vi "App - analyze RUS V6.vi"() -> ()   [LabVIEW 2021] (continued)
(VHz)"=0.0, "ω (Hz)"=0.0, "Γ (Hz)"=0.0, "φ (rad)"=0.0, "Q"=0.0, "Norm  Ampl"=0.0, "z∞ (V)"=0.0+0.0i, "4corners"={"z (-pi/2)"=0.0+0.0i, "z(inf)"=0.0+0.0i, "z (pi/2)"=0.0+0.0i, "z center"=0.0+0.0i, "z(0)"=0.0+0.0i, "radius"=0.0}}, "timestamp(min)"=1041.0333333313465, "timestamp"=timestamp(3493790283 s since 1904-01-01), "Magn Field(T)"=0.0}, {"temperature"=68.294, "lorentzian"={"A (VHz)"=0.0, "ω (Hz)"=0.0, "Γ (Hz)"=0.0, "φ (rad)"=0.0, "Q"=0.0, "Norm  Ampl"=0.0, "z∞ (V)"=0.0+0.0i, "4corners"={"z (-pi/2)"=0.0+0.0i, "z(inf)"=0.0+0.0i, "z (pi/2)"=0.0+0.0i, "z center"=0.0+0.0i, "z(0)"=0.0+0.0i, "radius"=0.0}}, "timestamp(min)"=1042.3500000014901, "timestamp"=timestamp(3493790362 s since 1904-01-01), "Magn Field(T)"=0.0}, {"temperature"=68.232, "lorentzian"={"A (VHz)"=0.0, "ω (Hz)"=0.0, "Γ (Hz)"=0.0, "φ (rad)"=0.0, "Q"=0.0, "Norm  Ampl"=0.0, "z∞ (V)"=0.0+0.0i, "4corners"={"z (-pi/2)"=0.0+0.0i, "z(inf)"=0.0+0.0i, "z (pi/2)"=0.0+0.0i, "z center"=0.0+0.0i, "z(0)"=0.0+0.0i, "radius"=0.0}}, "timestamp(min)"=1043.683333337307, "timestamp"=timestamp(3493790442 s since 1904-01-01), "Magn Field(T)"=0.0}, {"temperature"=68.168, "lorentzian"={"A (VHz)"=0.0, "ω (Hz)"=0.0, "Γ (Hz)"=0.0, "φ (rad)"=0.0, "Q"=0.0, "Norm  Ampl"=0.0, "z∞ (V)"=0.0+0.0i, "4corners"={"z (-pi/2)"=0.0+0.0i, "z(inf)"=0.0+0.0i, "z (pi/2)"=0.0+0.0i, "z center"=0.0+0.0i, "z(0)"=0.0+0.0i, "radius"=0.0}}, "timestamp(min)"=1045.0, "timestamp"=timestamp(3493790521 s since 1904-01-01), "Magn Field(T)"=0.0}, {"temperature"=68.111, "lorentzian"={"A (VHz)"=0.0, "ω (Hz)"=0.0, "Γ (Hz)"=0.0, "φ (rad)"=0.0, "Q"=0.0, "Norm  Ampl"=0.0, "z∞ (V)"=0.0+0.0i, "4corners"={"z (-pi/2)"=0.0+0.0i, "z(inf)"=0.0+0.0i, "z (pi/2)"=0.0+0.0i, "z center"=0.0+0.0i, "z(0)"=0.0+0.0i, "radius"=0.0}}, "timestamp(min)"=1046.3166666701436, "timestamp"=timestamp(3493790600 s since 1904-01-01), "Magn Field(T)"=0.0}, {"temperature"=68.048, "lorentzian"={"A (VHz)"=0.0, "ω (Hz)"=0.0, "Γ (Hz)"=0.0, "φ (rad)"=0.0, "Q"=0.0, "Norm  Ampl"=0.0, "z∞ (V)"=0.0+0.0i, "4corners"={"z (-pi/2)"=0.0+0.0i, "z(inf)"=0.0+0.0i, "z (pi/2)"=0.0+0.0i, "z center"=0.0+0.0i, "z(0)"=0.0+0.0i, "radius"=0.0}}, "timestamp(min)"=1047.6499999985099, "timestamp"=timestamp(3493790680 s since 1904-01-01), "Magn Field(T)"=0.0}, {"temperature"=67.989, "lorentzian"={"A (VHz)"=0.0, "ω (Hz)"=0.0, "Γ (Hz)"=0.0, "φ (rad)"=0.0, "Q"=0.0, "Norm  Ampl"=0.0, "z∞ (V)"=0.0+0.0i, "4corners"={"z (-pi/2)"=0.0+0.0i, "z(inf)"=0.0+0.0i, "z (pi/2)"=0.0+0.0i, "z center"=0.0+0.0i, "z(0)"=0.0+0.0i, "radius"=0.0}}, "timestamp(min)"=1048.9666666686535, "timestamp"=timestamp(3493790759 s since 1904-01-01), "Magn Field(T)"=0.0}, {"temperature"=67.927, "lorentzian"={"A (VHz)"=0.0, "ω (Hz)"=0.0, "Γ (Hz)"=0.0, "φ (rad)"=0.0, "Q"=0.0, "Norm  Ampl"=0.0, "z∞ (V)"=0.0+0.0i, "4corners"={"z (-pi/2)"=0.0+0.0i, "z(inf)"=0.0+0.0i, "z (pi/2)"=0.0+0.0i, "z center"=0.0+0.0i, "z(0)"=0.0+0.0i, "radius"=0.0}}, "timestamp(min)"=1050.2833333313465, "timestamp"=timestamp(3493790838 s since 1904-01-01), "Magn Field(T)"=0.0}, {"temperature"=67.865, "lorentzian"={"A (VHz)"=0.0, "ω (Hz)"=0.0, "Γ (Hz)"=0.0, "φ (rad)"=0.0, "Q"=0.0, "Norm  Ampl"=0.0, "z∞ (V)"=0.0+0.0i, "4corners"={"z (-pi/2)"=0.0+0.0i, "z(inf)"=0.0+0.0i, "z (pi/2)"=0.0+0.0i, "z center"=0.0+0.0i, "z(0)"=0.0+0.0i, "radius"=0.0}}, "timestamp(min)"=1051.6166666671634, "timestamp"=timestamp(3493790918 s since 1904-01-01), "Magn Field(T)"=0.0}, {"temperature"=67.806, "lorentzian"={"A (VHz)"=0.0, "ω (Hz)"=0.0, "Γ (Hz)"=0.0, "φ (rad)"=0.0, "Q"=0.0, "Norm  Ampl"=0.0, "z∞ (V)"=0.0+0.0i, "4corners"={"z (-pi/2)"=0.0+0.0i, "z(inf)"=0.0+0.0i, "z (pi/2)"=0.0+0.0i, "z center"=0.0+0.0i, "z(0)"=0.0+0.0i, "radius"=0.0}}, "timestamp(min)"=1052.933333337307, "timestamp"=timestamp(3493790997 s since 1904-01-01), "Magn Field(T)"=0.0}, {"temperature"=67.745, "lorentzian"={"A (VHz)"=0.0, "ω (Hz)"=0.0, "Γ (Hz)"=0.0, "φ (rad)"=0.0, "Q"=0.0, "Norm  Ampl"=0.0, "z∞ (V)"=0.0+0.0i, "4corners"={"z (-pi/2)"=0.0+0.0i, "z(inf)"=0.0+0.0i, "z (pi/2)"=0.0+0.0i, "z center"=0.0+0.0i, "z(0)"=0.0+0.0i, "radius"=0.0}}, "timestamp(min)"=1054.2666666656733, "timestamp"=timestamp(3493791077 s since 1904-01-01), "Magn Field(T)"=0.0}, {"temperature"=67.683, "lorentzian"={"A (VHz)"=0.0, "ω (Hz)"=0.0, "Γ (Hz)"=0.0, "φ (rad)"=0.0, "Q"=0.0, "Norm  Ampl"=0.0, "z∞ (V)"=0.0+0.0i, "4corners"={"z (-pi/2)"=0.0+0.0i, "z(inf)"=0.0+0.0i, "z (pi/2)"=0.0+0.0i, "z center"=0.0+0.0i, "z(0)"=0.0+0.0i, "radius"=0.0}}, "timestamp(min)"=1055.5833333358169, "timestamp"=timestamp(3493791156 s since 1904-01-01), "Magn Field(T)"=0.0}, {"temperature"=67.625, "lorentzian"={"A (VHz)"=0.0, "ω (Hz)"=0.0, "Γ (Hz)"=0.0, "φ (rad)"=0.0, "Q"=0.0, "Norm  Ampl"=0.0, "z∞ (V)"=0.0+0.0i, "4corners"={"z (-pi/2)"=0.0+0.0i, "z(inf)"=0.0+0.0i, "z (pi/2)"=0.0+0.0i, "z center"=0.0+0.0i, "z(0)"=0.0+0.0i, "radius"=0.0}}, "timestamp(min)"=1056.8999999985099, "timestamp"=timestamp(3493791235 s since 1904-01-01), "Magn Field(T)"=0.0}, {"temperature"=67.561, "lorentzian"={"A (VHz)"=0.0, "ω (Hz)"=0.0, "Γ (Hz)"=0.0, "φ (rad)"=0.0, "Q"=0.0, "Norm  Ampl"=0.0, "z∞ (V)"=0.0+0.0i, "4corners"={"z (-pi/2)"=0.0+0.0i, "z(inf)"=0.0+0.0i, "z (pi/2)"=0.0+0.0i, "z center"=0.0+0.0i, "z(0)"=0.0+0.0i, "radius"=0.0}}, "timestamp(min)"=1058.2333333343267, "timestamp"=timestamp(3493791315 s since 1904-01-01), "Magn Field(T)"=0.0}, {"temperature"=67.503, "lorentzian"={"A (VHz)"=0.0, "ω (Hz)"=0.0, "Γ (Hz)"=0.0, "φ (rad)"=0.0, "Q"=0.0, "Norm  Ampl"=0.0, "z∞ (V)"=0.0+0.0i, "4corners"={"z (-pi/2)"=0.0+0.0i, "z(inf)"=0.0+0.0i, "z (pi/2)"=0.0+0.0i, "z center"=0.0+0.0i, "z(0)"=0.0+0.0i, "radius"=0.0}}, "timestamp(min)"=1059.5500000044703, "timestamp"=timestamp(3493791394 s since 1904-01-01), "Magn Field(T)"=0.0}, {"temperature"=67.441, "lorentzian"={"A (VHz)"=0.0, "ω (Hz)"=0.0, "Γ (Hz)"=0.0, "φ (rad)"=0.0, "Q"=0.0, "Norm  Ampl"=0.0, "z∞ (V)"=0.0+0.0i, "4corners"={"z (-pi/2)"=0.0+0.0i, "z(inf)"=0.0+0.0i, "z (pi/2)"=0.0+0.0i, "z center"=0.0+0.0i, "z(0)"=0.0+0.0i, "radius"=0.0}}, "timestamp(min)"=1060.8666666671634, "timestamp"=timestamp(3493791473 s since 1904-01-01), "Magn Field(T)"=0.0}, {"temperature"=67.379, "lorentzian"={"A (VHz)"=0.0, "ω (Hz)"=0.0, "Γ (Hz)"=0.0, "φ (rad)"=0.0, "Q"=0.0, "Norm  Ampl"=0.0, "z∞ (V)"=0.0+0.0i, "4corners"={"z (-pi/2)"=0.0+0.0i, "z(inf)"=0.0+0.0i, "z (pi/2)"=0.0+0.0i, "z center"=0.0+0.0i, "z(0)"=0.0+0.0i, "radius"=0.0}}, "timestamp(min)"=1062.2000000029802, "timestamp"=timestamp(3493791553 s since 1904-01-01), "Magn Field(T)"=0.0}, {"temperature"=67.322, "lorentzian"={"A (VHz)"=0.0, "ω (Hz)"=0.0, "Γ (Hz)"=0.0, "φ (rad)"=0.0, "Q"=0.0, "Norm  Ampl"=0.0, "z∞ (V)"=0.0+0.0i, "4corners"={"z (-pi/2)"=0.0+0.0i, "z(inf)"=0.0+0.0i, "z (pi/2)"=0.0+0.0i, "z center"=0.0+0.0i, "z(0)"=0.0+0.0i, "radius"=0.0}}, "timestamp(min)"=1063.5166666656733, "timestamp"=timestamp(3493791632 s since 1904-01-01), "Magn Field(T)"=0.0}, {"temperature"=67.261, "lorentzian"={"A (VHz)"=0.0, "ω (Hz)"=0.0, "Γ (Hz)"=0.0, "φ (rad)"=0.0, "Q"=0.0, "Norm  Ampl"=0.0, "z∞ (V)"=0.0+0.0i, "4corners"={"z (-pi/2)"=0.0+0.0i, "z(inf)"=0.0+0.0i, "z (pi/2)"=0.0+0.0i, "z center"=0.0+0.0i, "z(0)"=0.0+0.0i, "radius"=0.0}}, "timestamp(min)"=1064.8333333358169, "timestamp"=timestamp(3493791711 s since 1904-01-01), "Magn Field(T)"=0.0}, {"temperature"=67.202, "lorentzian"={"A (VHz)"=0.0, "ω (Hz)"=0.0, "Γ (Hz)"=0.0, "φ (rad)"=0.0, "Q"=0.0, "Norm  Ampl"=0.0, "z∞ (V)"=0.0+0.0i, "4corners"={"z (-pi/2)"=0.0+0.0i, "z(inf)"=0.0+0.0i, "z (pi/2)"=0.0+0.0i, "z center"=0.0+0.0i, "z(0)"=0.0+0.0i, "radius"=0.0}}, "timestamp(min)"=1066.1666666641831, "timestamp"=timestamp(3493791791 s since 1904-01-01), "Magn Field(T)"=0.0}, {"temperature"=67.139, "lorentzian"={"A (VHz)"=0.0, "ω (Hz)"=0.0, "Γ (Hz)"=0.0, "φ (rad)"=0.0, "Q"=0.0, "Norm  Ampl"=0.0, "z∞ (V)"=0.0+0.0i, "4corners"={"z (-pi/2)"=0.0+0.0i, "z(inf)"=0.0+0.0i, "z (pi/2)"=0.0+0.0i, "z center"=0.0+0.0i, "z(0)"=0.0+0.0i, "radius"=0.0}}, "timestamp(min)"=1067.4833333343267, "timestamp"=timestamp(3493791870 s since 1904-01-01), "Magn Field(T)"=0.0}, {"temperature"=67.079, "lorentzian"={"A (VHz)"=0.0, "ω (Hz)"=0.0, "Γ (Hz)"=0.0, "φ (rad)"=0.0, "Q"=0.0, "Norm  Ampl"=0.0, "z∞ (V)"=0.0+0.0i, "4corners"={"z (-pi/2)"=0.0+0.0i, "z(inf)"=0.0+0.0i, "z (pi/2)"=0.0+0.0i, "z center"=0.0+0.0i, "z(0)"=0.0+0.0i, "radius"=0.0}}, "timestamp(min)"=1068.8000000044703, "timestamp"=timestamp(3493791949 s since 1904-01-01), "Magn Field(T)"=0.0}, {"temperature"=67.02, "lorentzian"={"A (VHz)"=0.0, "ω (Hz)"=0.0, "Γ (Hz)"=0.0, "φ (rad)"=0.0, "Q"=0.0, "Norm  Ampl"=0.0, "z∞ (V)"=0.0+0.0i, "4corners"={"z (-pi/2)"=0.0+0.0i, "z(inf)"=0.0+0.0i, "z (pi/2)"=0.0+0.0i, "z center"=0.0+0.0i, "z(0)"=0.0+0.0i, "radius"=0.0}}, "timestamp(min)"=1070.1333333328366, "timestamp"=timestamp(3493792029 s since 1904-01-01), "Magn Field(T)"=0.0}, {"temperature"=66.959, "lorentzian"={"A (VHz)"=0.0, "ω (Hz)"=0.0, "Γ (Hz)"=0.0, "φ (rad)"=0.0, "Q"=0.0, "Norm  Ampl"=0.0, "z∞ (V)"=0.0+0.0i, "4corners"={"z (-pi/2)"=0.0+0.0i, "z(inf)"=0.0+0.0i, "z (pi/2)"=0.0+0.0i, "z center"=0.0+0.0i, "z(0)"=0.0+0.0i, "radius"=0.0}}, "timestamp(min)"=1071.4500000029802, "timestamp"=timestamp(3493792108 s since 1904-01-01), "Magn Field(T)"=0.0}, {"temperature"=66.901, "lorentzian"={"A (VHz)"=0.0, "ω (Hz)"=0.0, "Γ (Hz)"=0.0, "φ (rad)"=0.0, "Q"=0.0, "Norm  Ampl"=0.0, "z∞ (V)"=0.0+0.0i, "4corners"={"z (-pi/2)"=0.0+0.0i, "z(inf)"=0.0+0.0i, "z (pi/2)"=0.0+0.0i, "z center"=0.0+0.0i, "z(0)"=0.0+0.0i, "radius"=0.0}}, "timestamp(min)"=1072.7666666656733, "timestamp"=timestamp(3493792187 s since 1904-01-01), "Magn Field(T)"=0.0}, {"temperature"=66.841, "lorentzian"={"A (VHz)"=0.0, "ω (Hz)"=0.0, "Γ (Hz)"=0.0, "φ (rad)"=0.0, "Q"=0.0, "Norm  Ampl"=0.0, "z∞ (V)"=0.0+0.0i, "4corners"={"z (-pi/2)"=0.0+0.0i, "z(inf)"=0.0+0.0i, "z (pi/2)"=0.0+0.0i, "z center"=0.0+0.0i, "z(0)"=0.0+0.0i, "radius"=0.0}}, "timestamp(min)"=1074.1000000014901, "timestamp"=timestamp(3493792267 s since 1904-01-01), "Magn Field(T)"=0.0}, {"temperature"=66.779, "lorentzian"={"A (VHz)"=0.0, "ω (Hz)"=0.0, "Γ (Hz)"=0.0, "φ (rad)"=0.0, "Q"=0.0, "Norm  Ampl"=0.0, "z∞ (V)"=0.0+0.0i, "4corners"={"z (-pi/2)"=0.0+0.0i, "z(inf)"=0.0+0.0i, "z (pi/2)"=0.0+0.0i, "z center"=0.0+0.0i, "z(0)"=0.0+0.0i, "radius"=0.0}}, "timestamp(min)"=1075.4166666641831, "timestamp"=timestamp(3493792346 s since 1904-01-01), "Magn Field(T)"=0.0}, {"temperature"=66.721, "lorentzian"={"A (VHz)"=0.0, "ω (Hz)"=0.0, "Γ (Hz)"=0.0, "φ (rad)"=0.0, "Q"=0.0, "Norm  Ampl"=0.0, "z∞ (V)"=0.0+0.0i, "4corners"={"z (-pi/2)"=0.0+0.0i, "z(inf)"=0.0+0.0i, "z (pi/2)"=0.0+0.0i, "z center"=0.0+0.0i, "z(0)"=0.0+0.0i, "radius"=0.0}}, "timestamp(min)"=1076.7333333343267, "timestamp"=timestamp(3493792425 s since 1904-01-01), "Magn Field(T)"=0.0}, {"temperature"=66.66, "lorentzian"={"A (VHz)"=0.0, "ω (Hz)"=0.0, "Γ (Hz)"=0.0, "φ (rad)"=0.0, "Q"=0.0, "Norm  Ampl"=0.0, "z∞ (V)"=0.0+0.0i, "4corners"={"z (-pi/2)"=0.0+0.0i, "z(inf)"=0.0+0.0i, "z (pi/2)"=0.0+0.0i, "z center"=0.0+0.0i, "z(0)"=0.0+0.0i, "radius"=0.0}}, "timestamp(min)"=1078.0666666701436, "timestamp"=timestamp(3493792505 s since 1904-01-01), "Magn Field(T)"=0.0}, {"temperature"=66.601, "lorentzian"={"A (VHz)"=0.0, "ω (Hz)"=0.0, "Γ (Hz)"=0.0, "φ (rad)"=0.0, "Q"=0.0, "Norm  Ampl"=0.0, "z∞ (V)"=0.0+0.0i, "4corners"={"z (-pi/2)"=0.0+0.0i, "z(inf)"=0.0+0.0i, "z (pi/2)"=0.0+0.0i, "z center"=0.0+0.0i, "z(0)"=0.0+0.0i, "radius"=0.0}}, "timestamp(min)"=1079.3833333328366, "timestamp"=timestamp(3493792584 s since 1904-01-01), "Magn Field(T)"=0.0}, {"temperature"=66.541, "lorentzian"={"A (VHz)"=0.0, "ω (Hz)"=0.0, "Γ (Hz)"=0.0, "φ (rad)"=0.0, "Q"=0.0, "Norm  Ampl"=0.0, "z∞ (V)"=0.0+0.0i, "4corners"={"z (-pi/2)"=0.0+0.0i, "z(inf)"=0.0+0.0i, "z (pi/2)"=0.0+0.0i, "z center"=0.0+0.0i, "z(0)"=0.0+0.0i, "radius"=0.0}}, "timestamp(min)"=1080.7166666686535, "timestamp"=timestamp(3493792664 s since 1904-01-01), "Magn Field(T)"=0.0}, {"temperature"=66.48, "lorentzian"={"A (VHz)"=0.0, "ω (Hz)"=0.0, "Γ (Hz)"=0.0, "φ (rad)"=0.0, "Q"=0.0, "Norm  Ampl"=0.0, "z∞ (V)"=0.0+0.0i, "4corners"={"z (-pi/2)"=0.0+0.0i, "z(inf)"=0.0+0.0i, "z (pi/2)"=0.0+0.0i, "z center"=0.0+0.0i, "z(0)"=0.0+0.0i, "radius"=0.0}}, "timestamp(min)"=1082.0333333313465, "timestamp"=timestamp(3493792743 s since 1904-01-01), "Magn Field(T)"=0.0}, {"temperature"=66.422, "lorentzian"={"A (VHz)"=0.0, "ω (Hz)"=0.0, "Γ (Hz)"=0.0, "φ (rad)"=0.0, "Q"=0.0, "Norm  Ampl"=0.0, "z∞ (V)"=0.0+0.0i, "4corners"={"z (-pi/2)"=0.0+0.0i, "z(inf)"=0.0+0.0i, "z (pi/2)"=0.0+0.0i, "z center"=0.0+0.0i, "z(0)"=0.0+0.0i, "radius"=0.0}}, "timestamp(min)"=1083.3500000014901, "timestamp"=timestamp(3493792822 s since 1904-01-01), "Magn Field(T)"=0.0}, {"temperature"=66.363, "lorentzian"={"A (VHz)"=0.0, "ω (Hz)"=0.0, "Γ (Hz)"=0.0, "φ (rad)"=0.0, "Q"=0.0, "Norm  Ampl"=0.0, "z∞ (V)"=0.0+0.0i, "4corners"={"z (-pi/2)"=0.0+0.0i, "z(inf)"=0.0+0.0i, "z (pi/2)"=0.0+0.0i, "z center"=0.0+0.0i, "z(0)"=0.0+0.0i, "radius"=0.0}}, "timestamp(min)"=1084.683333337307, "timestamp"=timestamp(3493792902 s since 1904-01-01), "Magn Field(T)"=0.0}, {"temperature"=66.302, "lorentzian"={"A (VHz)"=0.0, "ω (Hz)"=0.0, "Γ (Hz)"=0.0, "φ (rad)"=0.0, "Q"=0.0, "Norm  Ampl"=0.0, "z∞ (V)"=0.0+0.0i, "4corners"={"z (-pi/2)"=0.0+0.0i, "z(inf)"=0.0+0.0i, "z (pi/2)"=0.0+0.0i, "z center"=0.0+0.0i, "z(0)"=0.0+0.0i, "radius"=0.0}}, "timestamp(min)"=1086.0, "timestamp"=timestamp(3493792981 s since 1904-01-01), "Magn Field(T)"=0.0}, {"temperature"=66.244, "lorentzian"={"A (VHz)"=0.0, "ω (Hz)"=0.0, "Γ (Hz)"=0.0, "φ (rad)"=0.0, "Q"=0.0, "Norm  Ampl"=0.0, "z∞ (V)"=0.0+0.0i, "4corners"={"z (-pi/2)"=0.0+0.0i, "z(inf)"=0.0+0.0i, "z (pi/2)"=0.0+0.0i, "z center"=0.0+0.0i, "z(0)"=0.0+0.0i, "radius"=0.0}}, "timestamp(min)"=1087.3166666701436, "timestamp"=timestamp(3493793060 s since 1904-01-01), "Magn Field(T)"=0.0}, {"temperature"=66.182, "lorentzian"={"A (VHz)"=0.0, "ω (Hz)"=0.0, "Γ (Hz)"=0.0, "φ (rad)"=0.0, "Q"=0.0, "Norm  Ampl"=0.0, "z∞ (V)"=0.0+0.0i, "4corners"={"z (-pi/2)"=0.0+0.0i, "z(inf)"=0.0+0.0i, "z (pi/2)"=0.0+0.0i, "z center"=0.0+0.0i, "z(0)"=0.0+0.0i, "radius"=0.0}}, "timestamp(min)"=1088.6499999985099, "timestamp"=timestamp(3493793140 s since 1904-01-01), "Magn Field(T)"=0.0}, {"temperature"=66.124, "lorentzian"={"A (VHz)"=0.0, "ω (Hz)"=0.0, "Γ (Hz)"=0.0, "φ (rad)"=0.0, "Q"=0.0, "Norm  Ampl"=0.0, "z∞ (V)"=0.0+0.0i, "4corners"={"z (-pi/2)"=0.0+0.0i, "z(inf)"=0.0+0.0i, "z (pi/2)"=0.0+0.0i, "z center"=0.0+0.0i, "z(0)"=0.0+0.0i, "radius"=0.0}}, "timestamp(min)"=1089.9666666686535, "timestamp"=timestamp(3493793219 s since 1904-01-01), "Magn Field(T)"=0.0}, {"temperature"=66.063, "lorentzian"={"A (VHz)"=0.0, "ω (Hz)"=0.0, "Γ (Hz)"=0.0, "φ (rad)"=0.0, "Q"=0.0, "Norm  Ampl"=0.0, "z∞ (V)"=0.0+0.0i, "4corners"={"z (-pi/2)"=0.0+0.0i, "z(inf)"=0.0+0.0i, "z (pi/2)"=0.0+0.0i, "z center"=0.0+0.0i, "z(0)"=0.0+0.0i, "radius"=0.0}}, "timestamp(min)"=1091.3000000044703, "timestamp"=timestamp(3493793299 s since 1904-01-01), "Magn Field(T)"=0.0}, {"temperature"=66.006, "lorentzian"={"A (VHz)"=0.0, "ω (Hz)"=0.0, "Γ (Hz)"=0.0, "φ (rad)"=0.0, "Q"=0.0, "Norm  Ampl"=0.0, "z∞ (V)"=0.0+0.0i, "4corners"={"z (-pi/2)"=0.0+0.0i, "z(inf)"=0.0+0.0i, "z (pi/2)"=0.0+0.0i, "z center"=0.0+0.0i, "z(0)"=0.0+0.0i, "radius"=0.0}}, "timestamp(min)"=1092.6166666671634, "timestamp"=timestamp(3493793378 s since 1904-01-01), "Magn Field(T)"=0.0}, {"temperature"=65.947, "lorentzian"={"A (VHz)"=0.0, "ω (Hz)"=0.0, "Γ (Hz)"=0.0, "φ (rad)"=0.0, "Q"=0.0, "Norm  Ampl"=0.0, "z∞ (V)"=0.0+0.0i, "4corners"={"z (-pi/2)"=0.0+0.0i, "z(inf)"=0.0+0.0i, "z (pi/2)"=0.0+0.0i, "z center"=0.0+0.0i, "z(0)"=0.0+0.0i, "radius"=0.0}}, "timestamp(min)"=1093.933333337307, "timestamp"=timestamp(3493793457 s since 1904-01-01), "Magn Field(T)"=0.0}, {"temperature"=65.884, "lorentzian"={"A (VHz)"=0.0, "ω (Hz)"=0.0, "Γ (Hz)"=0.0, "φ (rad)"=0.0, "Q"=0.0, "Norm  Ampl"=0.0, "z∞ (V)"=0.0+0.0i, "4corners"={"z (-pi/2)"=0.0+0.0i, "z(inf)"=0.0+0.0i, "z (pi/2)"=0.0+0.0i, "z center"=0.0+0.0i, "z(0)"=0.0+0.0i, "radius"=0.0}}, "timestamp(min)"=1095.2666666656733, "timestamp"=timestamp(3493793537 s since 1904-01-01), "Magn Field(T)"=0.0}, {"temperature"=65.828, "lorentzian"={"A (VHz)"=0.0, "ω (Hz)"=0.0, "Γ (Hz)"=0.0, "φ (rad)"=0.0, "Q"=0.0, "Norm  Ampl"=0.0, "z∞ (V)"=0.0+0.0i, "4corners"={"z (-pi/2)"=0.0+0.0i, "z(inf)"=0.0+0.0i, "z (pi/2)"=0.0+0.0i, "z center"=0.0+0.0i, "z(0)"=0.0+0.0i, "radius"=0.0}}, "timestamp(min)"=1096.5833333358169, "timestamp"=timestamp(3493793616 s since 1904-01-01), "Magn Field(T)"=0.0}, {"temperature"=65.767, "lorentzian"={"A (VHz)"=0.0, "ω (Hz)"=0.0, "Γ (Hz)"=0.0, "φ (rad)"=0.0, "Q"=0.0, "Norm  Ampl"=0.0, "z∞ (V)"=0.0+0.0i, "4corners"={"z (-pi/2)"=0.0+0.0i, "z(inf)"=0.0+0.0i, "z (pi/2)"=0.0+0.0i, "z center"=0.0+0.0i, "z(0)"=0.0+0.0i, "radius"=0.0}}, "timestamp(min)"=1097.9166666641831, "timestamp"=timestamp(3493793696 s since 1904-01-01), "Magn Field(T)"=0.0}, {"temperature"=65.71, "lorentzian"={"A (VHz)"=0.0, "ω (Hz)"=0.0, "Γ (Hz)"=0.0, "φ (rad)"=0.0, "Q"=0.0, "Norm  Ampl"=0.0, "z∞ (V)"=0.0+0.0i, "4corners"={"z (-pi/2)"=0.0+0.0i, "z(inf)"=0.0+0.0i, "z (pi/2)"=0.0+0.0i, "z center"=0.0+0.0i, "z(0)"=0.0+0.0i, "radius"=0.0}}, "timestamp(min)"=1099.2333333343267, "timestamp"=timestamp(3493793775 s since 1904-01-01), "Magn Field(T)"=0.0}, {"temperature"=65.648, "lorentzian"={"A (VHz)"=0.0, "ω (Hz)"=0.0, "Γ (Hz)"=0.0, "φ (rad)"=0.0, "Q"=0.0, "Norm  Ampl"=0.0, "z∞ (V)"=0.0+0.0i, "4corners"={"z (-pi/2)"=0.0+0.0i, "z(inf)"=0.0+0.0i, "z (pi/2)"=0.0+0.0i, "z center"=0.0+0.0i, "z(0)"=0.0+0.0i, "radius"=0.0}}, "timestamp(min)"=1100.5500000044703, "timestamp"=timestamp(3493793854 s since 1904-01-01), "Magn Field(T)"=0.0}, {"temperature"=65.588, "lorentzian"={"A (VHz)"=0.0, "ω (Hz)"=0.0, "Γ (Hz)"=0.0, "φ (rad)"=0.0, "Q"=0.0, "Norm  Ampl"=0.0, "z∞ (V)"=0.0+0.0i, "4corners"={"z (-pi/2)"=0.0+0.0i, "z(inf)"=0.0+0.0i, "z (pi/2)"=0.0+0.0i, "z center"=0.0+0.0i, "z(0)"=0.0+0.0i, "radius"=0.0}}, "timestamp(min)"=1101.8833333328366, "timestamp"=timestamp(3493793934 s since 1904-01-01), "Magn Field(T)"=0.0}, {"temperature"=65.531, "lorentzian"={"A (VHz)"=0.0, "ω (Hz)"=0.0, "Γ (Hz)"=0.0, "φ (rad)"=0.0, "Q"=0.0, "Norm  Ampl"=0.0, "z∞ (V)"=0.0+0.0i, "4corners"={"z (-pi/2)"=0.0+0.0i, "z(inf)"=0.0+0.0i, "z (pi/2)"=0.0+0.0i, "z center"=0.0+0.0i, "z(0)"=0.0+0.0i, "radius"=0.0}}, "timestamp(min)"=1103.2000000029802, "timestamp"=timestamp(3493794013 s since 1904-01-01), "Magn Field(T)"=0.0}, {"temperature"=65.472, "lorentzian"={"A (VHz)"=0.0, "ω (Hz)"=0.0, "Γ (Hz)"=0.0, "φ (rad)"=0.0, "Q"=0.0, "Norm  Ampl"=0.0, "z∞ (V)"=0.0+0.0i, "4corners"={"z (-pi/2)"=0.0+0.0i, "z(inf)"=0.0+0.0i, "z (pi/2)"=0.0+0.0i, "z center"=0.0+0.0i, "z(0)"=0.0+0.0i, "radius"=0.0}}, "timestamp(min)"=1104.5166666656733, "timestamp"=timestamp(3493794092 s since 1904-01-01), "Magn Field(T)"=0.0}, {"temperature"=65.412, "lorentzian"={"A (VHz)"=0.0, "ω (Hz)"=0.0, "Γ (Hz)"=0.0, "φ (rad)"=0.0, "Q"=0.0, "Norm  Ampl"=0.0, "z∞ (V)"=0.0+0.0i, "4corners"={"z (-pi/2)"=0.0+0.0i, "z(inf)"=0.0+0.0i, "z (pi/2)"=0.0+0.0i, "z center"=0.0+0.0i, "z(0)"=0.0+0.0i, "radius"=0.0}}, "timestamp(min)"=1105.8500000014901, "timestamp"=timestamp(3493794172 s since 1904-01-01), "Magn Field(T)"=0.0}, {"temperature"=65.354, "lorentzian"={"A (VHz)"=0.0, "ω (Hz)"=0.0, "Γ (Hz)"=0.0, "φ (rad)"=0.0, "Q"=0.0, "Norm  Ampl"=0.0, "z∞ (V)"=0.0+0.0i, "4corners"={"z (-pi/2)"=0.0+0.0i, "z(inf)"=0.0+0.0i, "z (pi/2)"=0.0+0.0i, "z center"=0.0+0.0i, "z(0)"=0.0+0.0i, "radius"=0.0}}, "timestamp(min)"=1107.1666666641831, "timestamp"=timestamp(3493794251 s since 1904-01-01), "Magn Field(T)"=0.0}, {"temperature"=65.294, "lorentzian"={"A (VHz)"=0.0, "ω (Hz)"=0.0, "Γ (Hz)"=0.0, "φ (rad)"=0.0, "Q"=0.0, "Norm  Ampl"=0.0, "z∞ (V)"=0.0+0.0i, "4corners"={"z (-pi/2)"=0.0+0.0i, "z(inf)"=0.0+0.0i, "z (pi/2)"=0.0+0.0i, "z center"=0.0+0.0i, "z(0)"=0.0+0.0i, "radius"=0.0}}, "timestamp(min)"=1108.5, "timestamp"=timestamp(3493794331 s since 1904-01-01), "Magn Field(T)"=0.0}, {"temperature"=65.236, "lorentzian"={"A (VHz)"=0.0, "ω (Hz)"=0.0, "Γ (Hz)"=0.0, "φ (rad)"=0.0, "Q"=0.0, "Norm  Ampl"=0.0, "z∞ (V)"=0.0+0.0i, "4corners"={"z (-pi/2)"=0.0+0.0i, "z(inf)"=0.0+0.0i, "z (pi/2)"=0.0+0.0i, "z center"=0.0+0.0i, "z(0)"=0.0+0.0i, "radius"=0.0}}, "timestamp(min)"=1109.8166666701436, "timestamp"=timestamp(3493794410 s since 1904-01-01), "Magn Field(T)"=0.0}, {"temperature"=65.176, "lorentzian"={"A (VHz)"=0.0, "ω (Hz)"=0.0, "Γ (Hz)"=0.0, "φ (rad)"=0.0, "Q"=0.0, "Norm  Ampl"=0.0, "z∞ (V)"=0.0+0.0i, "4corners"={"z (-pi/2)"=0.0+0.0i, "z(inf)"=0.0+0.0i, "z (pi/2)"=0.0+0.0i, "z center"=0.0+0.0i, "z(0)"=0.0+0.0i, "radius"=0.0}}, "timestamp(min)"=1111.1333333328366, "timestamp"=timestamp(3493794489 s since 1904-01-01), "Magn Field(T)"=0.0}, {"temperature"=65.115, "lorentzian"={"A (VHz)"=0.0, "ω (Hz)"=0.0, "Γ (Hz)"=0.0, "φ (rad)"=0.0, "Q"=0.0, "Norm  Ampl"=0.0, "z∞ (V)"=0.0+0.0i, "4corners"={"z (-pi/2)"=0.0+0.0i, "z(inf)"=0.0+0.0i, "z (pi/2)"=0.0+0.0i, "z center"=0.0+0.0i, "z(0)"=0.0+0.0i, "radius"=0.0}}, "timestamp(min)"=1112.4666666686535, "timestamp"=timestamp(3493794569 s since 1904-01-01), "Magn Field(T)"=0.0}, {"temperature"=65.059, "lorentzian"={"A (VHz)"=0.0, "ω (Hz)"=0.0, "Γ (Hz)"=0.0, "φ (rad)"=0.0, "Q"=0.0, "Norm  Ampl"=0.0, "z∞ (V)"=0.0+0.0i, "4corners"={"z (-pi/2)"=0.0+0.0i, "z(inf)"=0.0+0.0i, "z (pi/2)"=0.0+0.0i, "z center"=0.0+0.0i, "z(0)"=0.0+0.0i, "radius"=0.0}}, "timestamp(min)"=1113.7833333313465, "timestamp"=timestamp(3493794648 s since 1904-01-01), "Magn Field(T)"=0.0}, {"temperature"=64.997, "lorentzian"={"A (VHz)"=0.0, "ω (Hz)"=0.0, "Γ (Hz)"=0.0, "φ (rad)"=0.0, "Q"=0.0, "Norm  Ampl"=0.0, "z∞ (V)"=0.0+0.0i, "4corners"={"z (-pi/2)"=0.0+0.0i, "z(inf)"=0.0+0.0i, "z (pi/2)"=0.0+0.0i, "z center"=0.0+0.0i, "z(0)"=0.0+0.0i, "radius"=0.0}}, "timestamp(min)"=1115.1166666671634, "timestamp"=timestamp(3493794728 s since 1904-01-01), "Magn Field(T)"=0.0}, {"temperature"=64.94, "lorentzian"={"A (VHz)"=0.0, "ω (Hz)"=0.0, "Γ (Hz)"=0.0, "φ (rad)"=0.0, "Q"=0.0, "Norm  Ampl"=0.0, "z∞ (V)"=0.0+0.0i, "4corners"={"z (-pi/2)"=0.0+0.0i, "z(inf)"=0.0+0.0i, "z (pi/2)"=0.0+0.0i, "z center"=0.0+0.0i, "z(0)"=0.0+0.0i, "radius"=0.0}}, "timestamp(min)"=1116.433333337307, "timestamp"=timestamp(3493794807 s since 1904-01-01), "Magn Field(T)"=0.0}, {"temperature"=64.883, "lorentzian"={"A (VHz)"=0.0, "ω (Hz)"=0.0, "Γ (Hz)"=0.0, "φ (rad)"=0.0, "Q"=0.0, "Norm  Ampl"=0.0, "z∞ (V)"=0.0+0.0i, "4corners"={"z (-pi/2)"=0.0+0.0i, "z(inf)"=0.0+0.0i, "z (pi/2)"=0.0+0.0i, "z center"=0.0+0.0i, "z(0)"=0.0+0.0i, "radius"=0.0}}, "timestamp(min)"=1117.75, "timestamp"=timestamp(3493794886 s since 1904-01-01), "Magn Field(T)"=0.0}, {"temperature"=64.821, "lorentzian"={"A (VHz)"=0.0, "ω (Hz)"=0.0, "Γ (Hz)"=0.0, "φ (rad)"=0.0, "Q"=0.0, "Norm  Ampl"=0.0, "z∞ (V)"=0.0+0.0i, "4corners"={"z (-pi/2)"=0.0+0.0i, "z(inf)"=0.0+0.0i, "z (pi/2)"=0.0+0.0i, "z center"=0.0+0.0i, "z(0)"=0.0+0.0i, "radius"=0.0}}, "timestamp(min)"=1119.0833333358169, "timestamp"=timestamp(3493794966 s since 1904-01-01), "Magn Field(T)"=0.0}, {"temperature"=64.764, "lorentzian"={"A (VHz)"=0.0, "ω (Hz)"=0.0, "Γ (Hz)"=0.0, "φ (rad)"=0.0, "Q"=0.0, "Norm  Ampl"=0.0, "z∞ (V)"=0.0+0.0i, "4corners"={"z (-pi/2)"=0.0+0.0i, "z(inf)"=0.0+0.0i, "z (pi/2)"=0.0+0.0i, "z center"=0.0+0.0i, "z(0)"=0.0+0.0i, "radius"=0.0}}, "timestamp(min)"=1120.3999999985099, "timestamp"=timestamp(3493795045 s since 1904-01-01), "Magn Field(T)"=0.0}, {"temperature"=64.703, "lorentzian"={"A (VHz)"=0.0, "ω (Hz)"=0.0, "Γ (Hz)"=0.0, "φ (rad)"=0.0, "Q"=0.0, "Norm  Ampl"=0.0, "z∞ (V)"=0.0+0.0i, "4corners"={"z (-pi/2)"=0.0+0.0i, "z(inf)"=0.0+0.0i, "z (pi/2)"=0.0+0.0i, "z center"=0.0+0.0i, "z(0)"=0.0+0.0i, "radius"=0.0}}, "timestamp(min)"=1121.7166666686535, "timestamp"=timestamp(3493795124 s since 1904-01-01), "Magn Field(T)"=0.0}, {"temperature"=64.649, "lorentzian"={"A (VHz)"=0.0, "ω (Hz)"=0.0, "Γ (Hz)"=0.0, "φ (rad)"=0.0, "Q"=0.0, "Norm  Ampl"=0.0, "z∞ (V)"=0.0+0.0i, "4corners"={"z (-pi/2)"=0.0+0.0i, "z(inf)"=0.0+0.0i, "z (pi/2)"=0.0+0.0i, "z center"=0.0+0.0i, "z(0)"=0.0+0.0i, "radius"=0.0}}, "timestamp(min)"=1123.0500000044703, "timestamp"=timestamp(3493795204 s since 1904-01-01), "Magn Field(T)"=0.0}, {"temperature"=64.588, "lorentzian"={"A (VHz)"=0.0, "ω (Hz)"=0.0, "Γ (Hz)"=0.0, "φ (rad)"=0.0, "Q"=0.0, "Norm  Ampl"=0.0, "z∞ (V)"=0.0+0.0i, "4corners"={"z (-pi/2)"=0.0+0.0i, "z(inf)"=0.0+0.0i, "z (pi/2)"=0.0+0.0i, "z center"=0.0+0.0i, "z(0)"=0.0+0.0i, "radius"=0.0}}, "timestamp(min)"=1124.3666666671634, "timestamp"=timestamp(3493795283 s since 1904-01-01), "Magn Field(T)"=0.0}, {"temperature"=64.527, "lorentzian"={"A (VHz)"=0.0, "ω (Hz)"=0.0, "Γ (Hz)"=0.0, "φ (rad)"=0.0, "Q"=0.0, "Norm  Ampl"=0.0, "z∞ (V)"=0.0+0.0i, "4corners"={"z (-pi/2)"=0.0+0.0i, "z(inf)"=0.0+0.0i, "z (pi/2)"=0.0+0.0i, "z center"=0.0+0.0i, "z(0)"=0.0+0.0i, "radius"=0.0}}, "timestamp(min)"=1125.7000000029802, "timestamp"=timestamp(3493795363 s since 1904-01-01), "Magn Field(T)"=0.0}, {"temperature"=64.473, "lorentzian"={"A (VHz)"=0.0, "ω (Hz)"=0.0, "Γ (Hz)"=0.0, "φ (rad)"=0.0, "Q"=0.0, "Norm  Ampl"=0.0, "z∞ (V)"=0.0+0.0i, "4corners"={"z (-pi/2)"=0.0+0.0i, "z(inf)"=0.0+0.0i, "z (pi/2)"=0.0+0.0i, "z center"=0.0+0.0i, "z(0)"=0.0+0.0i, "radius"=0.0}}, "timestamp(min)"=1127.0166666656733, "timestamp"=timestamp(3493795442 s since 1904-01-01), "Magn Field(T)"=0.0}, {"temperature"=64.413, "lorentzian"={"A (VHz)"=0.0, "ω (Hz)"=0.0, "Γ (Hz)"=0.0, "φ (rad)"=0.0, "Q"=0.0, "Norm  Ampl"=0.0, "z∞ (V)"=0.0+0.0i, "4corners"={"z (-pi/2)"=0.0+0.0i, "z(inf)"=0.0+0.0i, "z (pi/2)"=0.0+0.0i, "z center"=0.0+0.0i, "z(0)"=0.0+0.0i, "radius"=0.0}}, "timestamp(min)"=1128.3333333358169, "timestamp"=timestamp(3493795521 s since 1904-01-01), "Magn Field(T)"=0.0}, {"temperature"=64.354, "lorentzian"={"A (VHz)"=0.0, "ω (Hz)"=0.0, "Γ (Hz)"=0.0, "φ (rad)"=0.0, "Q"=0.0, "Norm  Ampl"=0.0, "z∞ (V)"=0.0+0.0i, "4corners"={"z (-pi/2)"=0.0+0.0i, "z(inf)"=0.0+0.0i, "z (pi/2)"=0.0+0.0i, "z center"=0.0+0.0i, "z(0)"=0.0+0.0i, "radius"=0.0}}, "timestamp(min)"=1129.6666666641831, "timestamp"=timestamp(3493795601 s since 1904-01-01), "Magn Field(T)"=0.0}, {"temperature"=64.292, "lorentzian"={"A (VHz)"=0.0, "ω (Hz)"=0.0, "Γ (Hz)"=0.0, "φ (rad)"=0.0, "Q"=0.0, "Norm  Ampl"=0.0, "z∞ (V)"=0.0+0.0i, "4corners"={"z (-pi/2)"=0.0+0.0i, "z(inf)"=0.0+0.0i, "z (pi/2)"=0.0+0.0i, "z center"=0.0+0.0i, "z(0)"=0.0+0.0i, "radius"=0.0}}, "timestamp(min)"=1130.9833333343267, "timestamp"=timestamp(3493795680 s since 1904-01-01), "Magn Field(T)"=0.0}, {"temperature"=64.234, "lorentzian"={"A (VHz)"=0.0, "ω (Hz)"=0.0, "Γ (Hz)"=0.0, "φ (rad)"=0.0, "Q"=0.0, "Norm  Ampl"=0.0, "z∞ (V)"=0.0+0.0i, "4corners"={"z (-pi/2)"=0.0+0.0i, "z(inf)"=0.0+0.0i, "z (pi/2)"=0.0+0.0i, "z center"=0.0+0.0i, "z(0)"=0.0+0.0i, "radius"=0.0}}, "timestamp(min)"=1132.3166666701436, "timestamp"=timestamp(3493795760 s since 1904-01-01), "Magn Field(T)"=0.0}, {"temperature"=64.177, "lorentzian"={"A (VHz)"=0.0, "ω (Hz)"=0.0, "Γ (Hz)"=0.0, "φ (rad)"=0.0, "Q"=0.0, "Norm  Ampl"=0.0, "z∞ (V)"=0.0+0.0i, "4corners"={"z (-pi/2)"=0.0+0.0i, "z(inf)"=0.0+0.0i, "z (pi/2)"=0.0+0.0i, "z center"=0.0+0.0i, "z(0)"=0.0+0.0i, "radius"=0.0}}, "timestamp(min)"=1133.6333333328366, "timestamp"=timestamp(3493795839 s since 1904-01-01), "Magn Field(T)"=0.0}, {"temperature"=64.117, "lorentzian"={"A (VHz)"=0.0, "ω (Hz)"=0.0, "Γ (Hz)"=0.0, "φ (rad)"=0.0, "Q"=0.0, "Norm  Ampl"=0.0, "z∞ (V)"=0.0+0.0i, "4corners"={"z (-pi/2)"=0.0+0.0i, "z(inf)"=0.0+0.0i, "z (pi/2)"=0.0+0.0i, "z center"=0.0+0.0i, "z(0)"=0.0+0.0i, "radius"=0.0}}, "timestamp(min)"=1134.9500000029802, "timestamp"=timestamp(3493795918 s since 1904-01-01), "Magn Field(T)"=0.0}, {"temperature"=64.06, "lorentzian"={"A (VHz)"=0.0, "ω (Hz)"=0.0, "Γ (Hz)"=0.0, "φ (rad)"=0.0, "Q"=0.0, "Norm  Ampl"=0.0, "z∞ (V)"=0.0+0.0i, "4corners"={"z (-pi/2)"=0.0+0.0i, "z(inf)"=0.0+0.0i, "z (pi/2)"=0.0+0.0i, "z center"=0.0+0.0i, "z(0)"=0.0+0.0i, "radius"=0.0}}, "timestamp(min)"=1136.2833333313465, "timestamp"=timestamp(3493795998 s since 1904-01-01), "Magn Field(T)"=0.0}, {"temperature"=64.001, "lorentzian"={"A (VHz)"=0.0, "ω (Hz)"=0.0, "Γ (Hz)"=0.0, "φ (rad)"=0.0, "Q"=0.0, "Norm  Ampl"=0.0, "z∞ (V)"=0.0+0.0i, "4corners"={"z (-pi/2)"=0.0+0.0i, "z(inf)"=0.0+0.0i, "z (pi/2)"=0.0+0.0i, "z center"=0.0+0.0i, "z(0)"=0.0+0.0i, "radius"=0.0}}, "timestamp(min)"=1137.6000000014901, "timestamp"=timestamp(3493796077 s since 1904-01-01), "Magn Field(T)"=0.0}, {"temperature"=63.941, "lorentzian"={"A (VHz)"=0.0, "ω (Hz)"=0.0, "Γ (Hz)"=0.0, "φ (rad)"=0.0, "Q"=0.0, "Norm  Ampl"=0.0, "z∞ (V)"=0.0+0.0i, "4corners"={"z (-pi/2)"=0.0+0.0i, "z(inf)"=0.0+0.0i, "z (pi/2)"=0.0+0.0i, "z center"=0.0+0.0i, "z(0)"=0.0+0.0i, "radius"=0.0}}, "timestamp(min)"=1138.9166666641831, "timestamp"=timestamp(3493796156 s since 1904-01-01), "Magn Field(T)"=0.0}, {"temperature"=63.884, "lorentzian"={"A (VHz)"=0.0, "ω (Hz)"=0.0, "Γ (Hz)"=0.0, "φ (rad)"=0.0, "Q"=0.0, "Norm  Ampl"=0.0, "z∞ (V)"=0.0+0.0i, "4corners"={"z (-pi/2)"=0.0+0.0i, "z(inf)"=0.0+0.0i, "z (pi/2)"=0.0+0.0i, "z center"=0.0+0.0i, "z(0)"=0.0+0.0i, "radius"=0.0}}, "timestamp(min)"=1140.25, "timestamp"=timestamp(3493796236 s since 1904-01-01), "Magn Field(T)"=0.0}, {"temperature"=63.822, "lorentzian"={"A (VHz)"=0.0, "ω (Hz)"=0.0, "Γ (Hz)"=0.0, "φ (rad)"=0.0, "Q"=0.0, "Norm  Ampl"=0.0, "z∞ (V)"=0.0+0.0i, "4corners"={"z (-pi/2)"=0.0+0.0i, "z(inf)"=0.0+0.0i, "z (pi/2)"=0.0+0.0i, "z center"=0.0+0.0i, "z(0)"=0.0+0.0i, "radius"=0.0}}, "timestamp(min)"=1141.5666666701436, "timestamp"=timestamp(3493796315 s since 1904-01-01), "Magn Field(T)"=0.0}, {"temperature"=63.767, "lorentzian"={"A (VHz)"=0.0, "ω (Hz)"=0.0, "Γ (Hz)"=0.0, "φ (rad)"=0.0, "Q"=0.0, "Norm  Ampl"=0.0, "z∞ (V)"=0.0+0.0i, "4corners"={"z (-pi/2)"=0.0+0.0i, "z(inf)"=0.0+0.0i, "z (pi/2)"=0.0+0.0i, "z center"=0.0+0.0i, "z(0)"=0.0+0.0i, "radius"=0.0}}, "timestamp(min)"=1142.8999999985099, "timestamp"=timestamp(3493796395 s since 1904-01-01), "Magn Field(T)"=0.0}, {"temperature"=63.708, "lorentzian"={"A (VHz)"=0.0, "ω (Hz)"=0.0, "Γ (Hz)"=0.0, "φ (rad)"=0.0, "Q"=0.0, "Norm  Ampl"=0.0, "z∞ (V)"=0.0+0.0i, "4corners"={"z (-pi/2)"=0.0+0.0i, "z(inf)"=0.0+0.0i, "z (pi/2)"=0.0+0.0i, "z center"=0.0+0.0i, "z(0)"=0.0+0.0i, "radius"=0.0}}, "timestamp(min)"=1144.2166666686535, "timestamp"=timestamp(3493796474 s since 1904-01-01), "Magn Field(T)"=0.0}, {"temperature"=63.646, "lorentzian"={"A (VHz)"=0.0, "ω (Hz)"=0.0, "Γ (Hz)"=0.0, "φ (rad)"=0.0, "Q"=0.0, "Norm  Ampl"=0.0, "z∞ (V)"=0.0+0.0i, "4corners"={"z (-pi/2)"=0.0+0.0i, "z(inf)"=0.0+0.0i, "z (pi/2)"=0.0+0.0i, "z center"=0.0+0.0i, "z(0)"=0.0+0.0i, "radius"=0.0}}, "timestamp(min)"=1145.5333333313465, "timestamp"=timestamp(3493796553 s since 1904-01-01), "Magn Field(T)"=0.0}, {"temperature"=63.59, "lorentzian"={"A (VHz)"=0.0, "ω (Hz)"=0.0, "Γ (Hz)"=0.0, "φ (rad)"=0.0, "Q"=0.0, "Norm  Ampl"=0.0, "z∞ (V)"=0.0+0.0i, "4corners"={"z (-pi/2)"=0.0+0.0i, "z(inf)"=0.0+0.0i, "z (pi/2)"=0.0+0.0i, "z center"=0.0+0.0i, "z(0)"=0.0+0.0i, "radius"=0.0}}, "timestamp(min)"=1146.8666666671634, "timestamp"=timestamp(3493796633 s since 1904-01-01), "Magn Field(T)"=0.0}, {"temperature"=63.532, "lorentzian"={"A (VHz)"=0.0, "ω (Hz)"=0.0, "Γ (Hz)"=0.0, "φ (rad)"=0.0, "Q"=0.0, "Norm  Ampl"=0.0, "z∞ (V)"=0.0+0.0i, "4corners"={"z (-pi/2)"=0.0+0.0i, "z(inf)"=0.0+0.0i, "z (pi/2)"=0.0+0.0i, "z center"=0.0+0.0i, "z(0)"=0.0+0.0i, "radius"=0.0}}, "timestamp(min)"=1148.183333337307, "timestamp"=timestamp(3493796712 s since 1904-01-01), "Magn Field(T)"=0.0}, {"temperature"=63.472, "lorentzian"={"A (VHz)"=0.0, "ω (Hz)"=0.0, "Γ (Hz)"=0.0, "φ (rad)"=0.0, "Q"=0.0, "Norm  Ampl"=0.0, "z∞ (V)"=0.0+0.0i, "4corners"={"z (-pi/2)"=0.0+0.0i, "z(inf)"=0.0+0.0i, "z (pi/2)"=0.0+0.0i, "z center"=0.0+0.0i, "z(0)"=0.0+0.0i, "radius"=0.0}}, "timestamp(min)"=1149.5, "timestamp"=timestamp(3493796791 s since 1904-01-01), "Magn Field(T)"=0.0}, {"temperature"=63.413, "lorentzian"={"A (VHz)"=0.0, "ω (Hz)"=0.0, "Γ (Hz)"=0.0, "φ (rad)"=0.0, "Q"=0.0, "Norm  Ampl"=0.0, "z∞ (V)"=0.0+0.0i, "4corners"={"z (-pi/2)"=0.0+0.0i, "z(inf)"=0.0+0.0i, "z (pi/2)"=0.0+0.0i, "z center"=0.0+0.0i, "z(0)"=0.0+0.0i, "radius"=0.0}}, "timestamp(min)"=1150.8333333358169, "timestamp"=timestamp(3493796871 s since 1904-01-01), "Magn Field(T)"=0.0}, {"temperature"=63.355, "lorentzian"={"A (VHz)"=0.0, "ω (Hz)"=0.0, "Γ (Hz)"=0.0, "φ (rad)"=0.0, "Q"=0.0, "Norm  Ampl"=0.0, "z∞ (V)"=0.0+0.0i, "4corners"={"z (-pi/2)"=0.0+0.0i, "z(inf)"=0.0+0.0i, "z (pi/2)"=0.0+0.0i, "z center"=0.0+0.0i, "z(0)"=0.0+0.0i, "radius"=0.0}}, "timestamp(min)"=1152.1499999985099, "timestamp"=timestamp(3493796950 s since 1904-01-01), "Magn Field(T)"=0.0}, {"temperature"=63.298, "lorentzian"={"A (VHz)"=0.0, "ω (Hz)"=0.0, "Γ (Hz)"=0.0, "φ (rad)"=0.0, "Q"=0.0, "Norm  Ampl"=0.0, "z∞ (V)"=0.0+0.0i, "4corners"={"z (-pi/2)"=0.0+0.0i, "z(inf)"=0.0+0.0i, "z (pi/2)"=0.0+0.0i, "z center"=0.0+0.0i, "z(0)"=0.0+0.0i, "radius"=0.0}}, "timestamp(min)"=1153.4833333343267, "timestamp"=timestamp(3493797030 s since 1904-01-01), "Magn Field(T)"=0.0}, {"temperature"=63.239, "lorentzian"={"A (VHz)"=0.0, "ω (Hz)"=0.0, "Γ (Hz)"=0.0, "φ (rad)"=0.0, "Q"=0.0, "Norm  Ampl"=0.0, "z∞ (V)"=0.0+0.0i, "4corners"={"z (-pi/2)"=0.0+0.0i, "z(inf)"=0.0+0.0i, "z (pi/2)"=0.0+0.0i, "z center"=0.0+0.0i, "z(0)"=0.0+0.0i, "radius"=0.0}}, "timestamp(min)"=1154.8000000044703, "timestamp"=timestamp(3493797109 s since 1904-01-01), "Magn Field(T)"=0.0}, {"temperature"=63.178, "lorentzian"={"A (VHz)"=0.0, "ω (Hz)"=0.0, "Γ (Hz)"=0.0, "φ (rad)"=0.0, "Q"=0.0, "Norm  Ampl"=0.0, "z∞ (V)"=0.0+0.0i, "4corners"={"z (-pi/2)"=0.0+0.0i, "z(inf)"=0.0+0.0i, "z (pi/2)"=0.0+0.0i, "z center"=0.0+0.0i, "z(0)"=0.0+0.0i, "radius"=0.0}}, "timestamp(min)"=1156.1166666671634, "timestamp"=timestamp(3493797188 s since 1904-01-01), "Magn Field(T)"=0.0}, {"temperature"=63.123, "lorentzian"={"A (VHz)"=0.0, "ω (Hz)"=0.0, "Γ (Hz)"=0.0, "φ (rad)"=0.0, "Q"=0.0, "Norm  Ampl"=0.0, "z∞ (V)"=0.0+0.0i, "4corners"={"z (-pi/2)"=0.0+0.0i, "z(inf)"=0.0+0.0i, "z (pi/2)"=0.0+0.0i, "z center"=0.0+0.0i, "z(0)"=0.0+0.0i, "radius"=0.0}}, "timestamp(min)"=1157.4500000029802, "timestamp"=timestamp(3493797268 s since 1904-01-01), "Magn Field(T)"=0.0}, {"temperature"=63.063, "lorentzian"={"A (VHz)"=0.0, "ω (Hz)"=0.0, "Γ (Hz)"=0.0, "φ (rad)"=0.0, "Q"=0.0, "Norm  Ampl"=0.0, "z∞ (V)"=0.0+0.0i, "4corners"={"z (-pi/2)"=0.0+0.0i, "z(inf)"=0.0+0.0i, "z (pi/2)"=0.0+0.0i, "z center"=0.0+0.0i, "z(0)"=0.0+0.0i, "radius"=0.0}}, "timestamp(min)"=1158.7666666656733, "timestamp"=timestamp(3493797347 s since 1904-01-01), "Magn Field(T)"=0.0}, {"temperature"=63.004, "lorentzian"={"A (VHz)"=0.0, "ω (Hz)"=0.0, "Γ (Hz)"=0.0, "φ (rad)"=0.0, "Q"=0.0, "Norm  Ampl"=0.0, "z∞ (V)"=0.0+0.0i, "4corners"={"z (-pi/2)"=0.0+0.0i, "z(inf)"=0.0+0.0i, "z (pi/2)"=0.0+0.0i, "z center"=0.0+0.0i, "z(0)"=0.0+0.0i, "radius"=0.0}}, "timestamp(min)"=1160.1000000014901, "timestamp"=timestamp(3493797427 s since 1904-01-01), "Magn Field(T)"=0.0}, {"temperature"=62.948, "lorentzian"={"A (VHz)"=0.0, "ω (Hz)"=0.0, "Γ (Hz)"=0.0, "φ (rad)"=0.0, "Q"=0.0, "Norm  Ampl"=0.0, "z∞ (V)"=0.0+0.0i, "4corners"={"z (-pi/2)"=0.0+0.0i, "z(inf)"=0.0+0.0i, "z (pi/2)"=0.0+0.0i, "z center"=0.0+0.0i, "z(0)"=0.0+0.0i, "radius"=0.0}}, "timestamp(min)"=1161.4166666641831, "timestamp"=timestamp(3493797506 s since 1904-01-01), "Magn Field(T)"=0.0}, {"temperature"=62.886, "lorentzian"={"A (VHz)"=0.0, "ω (Hz)"=0.0, "Γ (Hz)"=0.0, "φ (rad)"=0.0, "Q"=0.0, "Norm  Ampl"=0.0, "z∞ (V)"=0.0+0.0i, "4corners"={"z (-pi/2)"=0.0+0.0i, "z(inf)"=0.0+0.0i, "z (pi/2)"=0.0+0.0i, "z center"=0.0+0.0i, "z(0)"=0.0+0.0i, "radius"=0.0}}, "timestamp(min)"=1162.7333333343267, "timestamp"=timestamp(3493797585 s since 1904-01-01), "Magn Field(T)"=0.0}, {"temperature"=62.828, "lorentzian"={"A (VHz)"=0.0, "ω (Hz)"=0.0, "Γ (Hz)"=0.0, "φ (rad)"=0.0, "Q"=0.0, "Norm  Ampl"=0.0, "z∞ (V)"=0.0+0.0i, "4corners"={"z (-pi/2)"=0.0+0.0i, "z(inf)"=0.0+0.0i, "z (pi/2)"=0.0+0.0i, "z center"=0.0+0.0i, "z(0)"=0.0+0.0i, "radius"=0.0}}, "timestamp(min)"=1164.0666666701436, "timestamp"=timestamp(3493797665 s since 1904-01-01), "Magn Field(T)"=0.0}, {"temperature"=62.769, "lorentzian"={"A (VHz)"=0.0, "ω (Hz)"=0.0, "Γ (Hz)"=0.0, "φ (rad)"=0.0, "Q"=0.0, "Norm  Ampl"=0.0, "z∞ (V)"=0.0+0.0i, "4corners"={"z (-pi/2)"=0.0+0.0i, "z(inf)"=0.0+0.0i, "z (pi/2)"=0.0+0.0i, "z center"=0.0+0.0i, "z(0)"=0.0+0.0i, "radius"=0.0}}, "timestamp(min)"=1165.3833333328366, "timestamp"=timestamp(3493797744 s since 1904-01-01), "Magn Field(T)"=0.0}, {"temperature"=62.713, "lorentzian"={"A (VHz)"=0.0, "ω (Hz)"=0.0, "Γ (Hz)"=0.0, "φ (rad)"=0.0, "Q"=0.0, "Norm  Ampl"=0.0, "z∞ (V)"=0.0+0.0i, "4corners"={"z (-pi/2)"=0.0+0.0i, "z(inf)"=0.0+0.0i, "z (pi/2)"=0.0+0.0i, "z center"=0.0+0.0i, "z(0)"=0.0+0.0i, "radius"=0.0}}, "timestamp(min)"=1166.7000000029802, "timestamp"=timestamp(3493797823 s since 1904-01-01), "Magn Field(T)"=0.0}, {"temperature"=62.654, "lorentzian"={"A (VHz)"=0.0, "ω (Hz)"=0.0, "Γ (Hz)"=0.0, "φ (rad)"=0.0, "Q"=0.0, "Norm  Ampl"=0.0, "z∞ (V)"=0.0+0.0i, "4corners"={"z (-pi/2)"=0.0+0.0i, "z(inf)"=0.0+0.0i, "z (pi/2)"=0.0+0.0i, "z center"=0.0+0.0i, "z(0)"=0.0+0.0i, "radius"=0.0}}, "timestamp(min)"=1168.0333333313465, "timestamp"=timestamp(3493797903 s since 1904-01-01), "Magn Field(T)"=0.0}, {"temperature"=62.592, "lorentzian"={"A (VHz)"=0.0, "ω (Hz)"=0.0, "Γ (Hz)"=0.0, "φ (rad)"=0.0, "Q"=0.0, "Norm  Ampl"=0.0, "z∞ (V)"=0.0+0.0i, "4corners"={"z (-pi/2)"=0.0+0.0i, "z(inf)"=0.0+0.0i, "z (pi/2)"=0.0+0.0i, "z center"=0.0+0.0i, "z(0)"=0.0+0.0i, "radius"=0.0}}, "timestamp(min)"=1169.3500000014901, "timestamp"=timestamp(3493797982 s since 1904-01-01), "Magn Field(T)"=0.0}, {"temperature"=62.537, "lorentzian"={"A (VHz)"=0.0, "ω (Hz)"=0.0, "Γ (Hz)"=0.0, "φ (rad)"=0.0, "Q"=0.0, "Norm  Ampl"=0.0, "z∞ (V)"=0.0+0.0i, "4corners"={"z (-pi/2)"=0.0+0.0i, "z(inf)"=0.0+0.0i, "z (pi/2)"=0.0+0.0i, "z center"=0.0+0.0i, "z(0)"=0.0+0.0i, "radius"=0.0}}, "timestamp(min)"=1170.683333337307, "timestamp"=timestamp(3493798062 s since 1904-01-01), "Magn Field(T)"=0.0}, {"temperature"=62.48, "lorentzian"={"A (VHz)"=0.0, "ω (Hz)"=0.0, "Γ (Hz)"=0.0, "φ (rad)"=0.0, "Q"=0.0, "Norm  Ampl"=0.0, "z∞ (V)"=0.0+0.0i, "4corners"={"z (-pi/2)"=0.0+0.0i, "z(inf)"=0.0+0.0i, "z (pi/2)"=0.0+0.0i, "z center"=0.0+0.0i, "z(0)"=0.0+0.0i, "radius"=0.0}}, "timestamp(min)"=1172.0, "timestamp"=timestamp(3493798141 s since 1904-01-01), "Magn Field(T)"=0.0}, {"temperature"=62.42, "lorentzian"={"A (VHz)"=0.0, "ω (Hz)"=0.0, "Γ (Hz)"=0.0, "φ (rad)"=0.0, "Q"=0.0, "Norm  Ampl"=0.0, "z∞ (V)"=0.0+0.0i, "4corners"={"z (-pi/2)"=0.0+0.0i, "z(inf)"=0.0+0.0i, "z (pi/2)"=0.0+0.0i, "z center"=0.0+0.0i, "z(0)"=0.0+0.0i, "radius"=0.0}}, "timestamp(min)"=1173.3166666701436, "timestamp"=timestamp(3493798220 s since 1904-01-01), "Magn Field(T)"=0.0}, {"temperature"=62.361, "lorentzian"={"A (VHz)"=0.0, "ω (Hz)"=0.0, "Γ (Hz)"=0.0, "φ (rad)"=0.0, "Q"=0.0, "Norm  Ampl"=0.0, "z∞ (V)"=0.0+0.0i, "4corners"={"z (-pi/2)"=0.0+0.0i, "z(inf)"=0.0+0.0i, "z (pi/2)"=0.0+0.0i, "z center"=0.0+0.0i, "z(0)"=0.0+0.0i, "radius"=0.0}}, "timestamp(min)"=1174.6499999985099, "timestamp"=timestamp(3493798300 s since 1904-01-01), "Magn Field(T)"=0.0}, {"temperature"=62.301, "lorentzian"={"A (VHz)"=0.0, "ω (Hz)"=0.0, "Γ (Hz)"=0.0, "φ (rad)"=0.0, "Q"=0.0, "Norm  Ampl"=0.0, "z∞ (V)"=0.0+0.0i, "4corners"={"z (-pi/2)"=0.0+0.0i, "z(inf)"=0.0+0.0i, "z (pi/2)"=0.0+0.0i, "z center"=0.0+0.0i, "z(0)"=0.0+0.0i, "radius"=0.0}}, "timestamp(min)"=1175.9666666686535, "timestamp"=timestamp(3493798379 s since 1904-01-01), "Magn Field(T)"=0.0}, {"temperature"=62.245, "lorentzian"={"A (VHz)"=0.0, "ω (Hz)"=0.0, "Γ (Hz)"=0.0, "φ (rad)"=0.0, "Q"=0.0, "Norm  Ampl"=0.0, "z∞ (V)"=0.0+0.0i, "4corners"={"z (-pi/2)"=0.0+0.0i, "z(inf)"=0.0+0.0i, "z (pi/2)"=0.0+0.0i, "z center"=0.0+0.0i, "z(0)"=0.0+0.0i, "radius"=0.0}}, "timestamp(min)"=1177.3000000044703, "timestamp"=timestamp(3493798459 s since 1904-01-01), "Magn Field(T)"=0.0}, {"temperature"=62.184, "lorentzian"={"A (VHz)"=0.0, "ω (Hz)"=0.0, "Γ (Hz)"=0.0, "φ (rad)"=0.0, "Q"=0.0, "Norm  Ampl"=0.0, "z∞ (V)"=0.0+0.0i, "4corners"={"z (-pi/2)"=0.0+0.0i, "z(inf)"=0.0+0.0i, "z (pi/2)"=0.0+0.0i, "z center"=0.0+0.0i, "z(0)"=0.0+0.0i, "radius"=0.0}}, "timestamp(min)"=1178.6166666671634, "timestamp"=timestamp(3493798538 s since 1904-01-01), "Magn Field(T)"=0.0}, {"temperature"=62.127, "lorentzian"={"A 
